vi "Close.vi"(8 "error in (no error)":errorcluster, 11 "Data in":refnum<class "OnChangeNotifier_SGL.lvclass">) -> (0 "error out":errorcluster, 3 "Data out":refnum<class "OnChangeNotifier_SGL.lvclass">)   [LabVIEW 2021, in "OnChangeNotifier_SGL.lvclass"]
doc: "Abstract Data Classes 2.1.1.13\nTim Streeter - TSA\nCopyright (c) 2025, TSA"
uses:
  OnChangeNotifier_SGL.lvclass
  OnChangeNotifier_SGL.lvclass/OnChangeNotifier_SGL.ctl
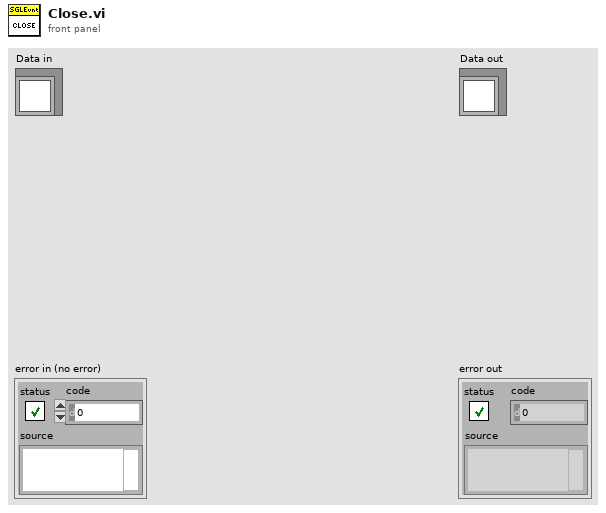
[diagram p1: front panel]
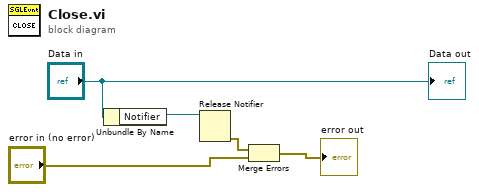
[diagram p0: block diagram]
diagram:
  n1 = Unbundle By Name("Data in") -> ("Notifier"=w2:refnum<notifier>)
  n2 = Release Notifier(notifier=w2) -> (error out=w1:errorcluster)  [unwired: 2 in, 2 out]
  n3 = Merge Errors(w1, "error in (no error)") -> (→"error out":errorcluster)
  "Data out" <- "Data in"
